vi "Read OpCfg from GXML File.vi"(8 "error in (no error)":errorcluster, 11 "Path":path) -> (0 "error out":errorcluster, 2 "Found":bool, 5 "Version String":string)   [LabVIEW 2015, in "Tool Cfg.lvlib"]
uses:
  Tool Cfg.lvlib
  _Tool Operation Config Cluster--typedef.ctl
  ConfigGLOB.vi
  <vilib>/NI/GXML/GXML.lvlib
panel:
  out "XML String Out":string
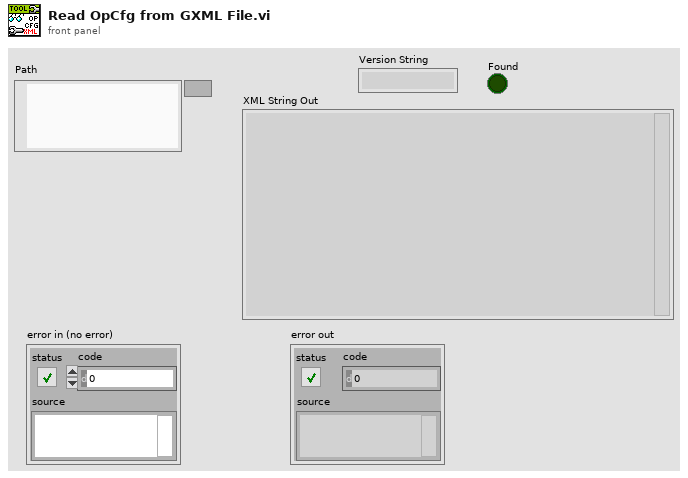
[diagram p1: front panel]
types:
  T1 = typedef "Tool Cfg.lvlib/_Tool Operation Config Cluster--typedef.ctl" = cluster{"Use Tool Cfg":bool, "Use Tool Cal":bool, "Fake Data?":bool, "Mode":i16, "Array Subset Length":i16, "nArrays to Read":i16, "Full Array Read Length":i16, "nSubarrays/Sensor":i16}
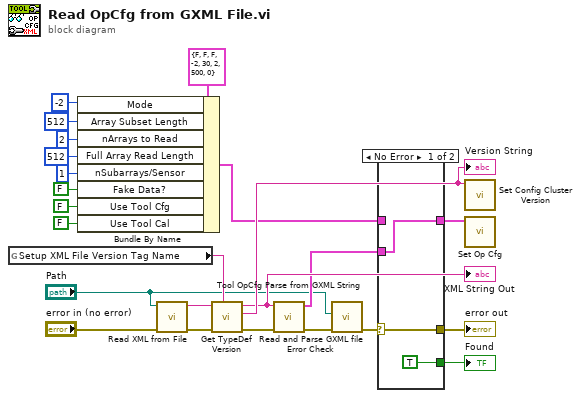
[diagram p0: block diagram]
diagram:
  n1 = global read "ConfigGLOB.vi" "Setup XML File Version Tag Name"() -> (w9:string)
  n2 = Bundle By Name(cluster=T1 {"Use Tool Cfg"=FALSE, "Use Tool Cal"=FALSE, "Fake Data?"=FALSE, "Mode"=-2, "Array Subset Length"=30, "nArrays to Read"=2, "Full Array Read Length"=500, "nSubarrays/Sensor"=0} ("_Tool Operation Config Cluster--typedef"), "Mode"=i16 -2, "Array Subset Length"=i16 512 ("Array Type"), "nArrays to Read"=i16 2, "Full Array Read Length"=i16 512, "nSubarrays/Sensor"=i16 1 ("Full Array Read Length"), "Fake Data?"=FALSE, "Use Tool Cfg"=FALSE, "Use Tool Cal"=FALSE) -> (w4:T1)
  n3 = call <vilib>:"Read XML from File.vi"("error in"="error in (no error)", "XML File Path"="Path") -> ("error out"=w23:errorcluster, "XML String Out"=w22:string)  [unwired: 8 in]
  n4 = call <vilib>:"Get TypeDef Version.vi"("Version Tag Name"=w9, "error in"=w23, "XML String In"=w22) -> ("error out"=w21:errorcluster, "Version String"=w11:string, "XML String Out"=w10:string)  [unwired: 6 in]
  "XML String Out" <- w10
  "Version String" <- w11
  n5 = call "Tool OpCfg Parse from GXML String.vi"("error in (no error)"=w21, "XML String In"=w10) -> ("error out"=w8:errorcluster, "Tool Op Cfg Cluster out"=w6:T1)  [unwired: 8 in]
  n6 = call "Read and Parse GXML file Error Check.vi"("error in (no error)"=w8, "Path"="Path") -> ("error out"=w7:errorcluster)  [unwired: 9 in]
  n7 = case shown="No Error" w7 {
    selector: w7 -> [w25 w28]
    tunnel: w6 -> [w27 _]
    tunnel: [w27 w29] -> w5
    tunnel: w4 -> [_ w29]
    tunnel: [TRUE _] -> w3
    tunnel: [w25 w28] -> w2
    frame No Error {
    }
    frame Error {
    }
  }
  "error out" <- w2
  "Found" <- w3
  n8 = call "Set Config Cluster Version.vi"("Config Cluster Version"=w11) -> ()  [unwired: 11 in]
  n9 = call "Set Op Cfg.vi"("Tool Operation Config"=w5) -> ()  [unwired: 11 in]
